vi "TestObjective_init.vi"(8 "error in (no error)":errorcluster, 10 "GameRef":refnum<data-value>, 11 "TestObjetive in":refnum<class "TestObjetive.lvclass">) -> (0 "error out":errorcluster, 3 "TestObjetive out":refnum<class "TestObjetive.lvclass">)   [LabVIEW 2023, in "TestObjetive.lvclass"]
uses:
  TestObjetive.lvclass
  Game_class/Game.lvclass
  TestObjetive.lvclass/TestObjetive.ctl
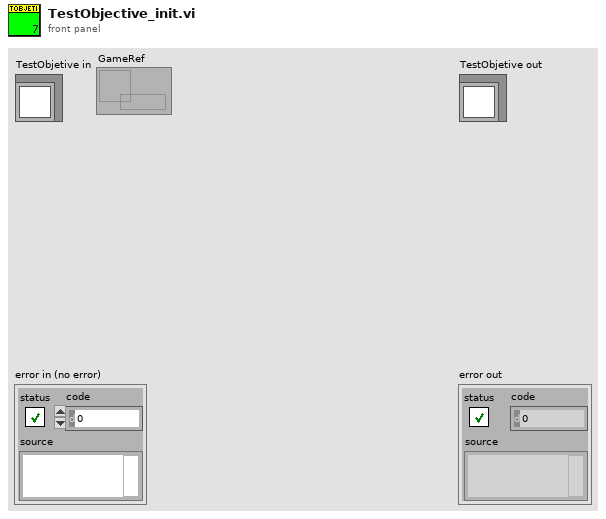
[diagram p1: front panel]
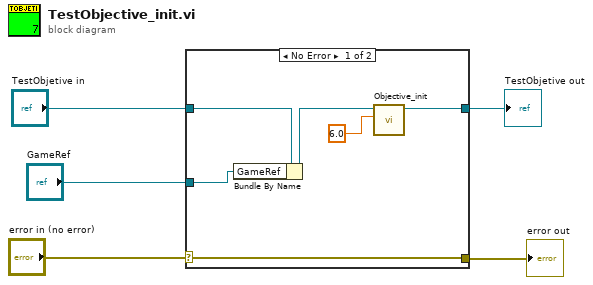
[diagram p0: block diagram]
diagram:
  n1 = case shown="No Error" "error in (no error)" {
    selector: "error in (no error)" -> [w11 w13]
    tunnel: [w11 w13] -> w4
    tunnel: [w8 w12] -> w2
    tunnel: "TestObjetive in" -> [w10 w12]
    tunnel: "GameRef" -> [w6 _]
    frame No Error {
      n2 = Bundle By Name(cluster=w10, "GameRef"=w6) -> (w9:refnum<class "TestObjetive.lvclass">)
      n3 = call-dynamic "Objective_init.vi"("maxEval"=6.0, "Objective in"=w9) -> ("Objective out"=w8:refnum<class "TestObjetive.lvclass">)  [unwired: 8 in, 1 out]
    }
    frame Error {
    }
  }
  "error out" <- w4
  "TestObjetive out" <- w2
